vi "GetIMFreqs.vi"(6 "Legacy (f)?":bool, 8 "error in (no error)":errorcluster) -> (0 "error out":errorcluster, 2 "IMFreqs":dbl[](array[numeric]) format="%.2f")   [LabVIEW 2011]
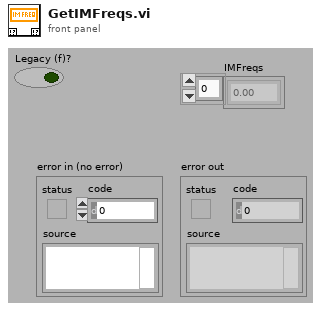
[diagram p1: front panel]
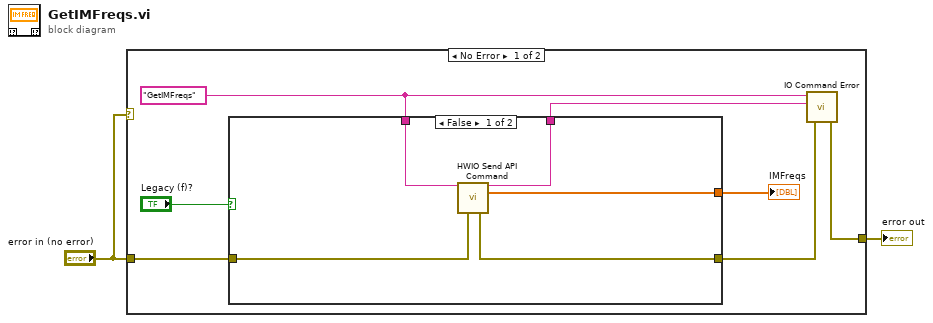
[diagram p0: block diagram]
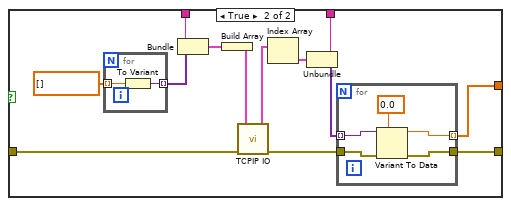
[diagram p2: hidden frame]
diagram:
  n1 = case shown="No Error" "error in (no error)" {
    tunnel: "error in (no error)" -> [w8 w35]
    tunnel: [w5 w35] -> w2
    frame No Error {
      w7 = "GetIMFreqs"
      n2 = case shown="False" "Legacy (f)?" {
        tunnel: [w12 w23] -> w9
        tunnel: w8 -> [w14 w21]
        tunnel: w7 -> [w10 w20]
        tunnel: [w13 w19] -> w6
        tunnel: [w11 w18] -> w4
        frame False {
          n3 = call "HWIO Send API Command.vi"("Action"=w10, "error in (no error)"=w14) -> ("Action out"=w11:string, "Double out"=w12:dbl[], "error out"=w13:errorcluster)  [unwired: 6 in, 5 out]
        }
        frame True {
          n4 = for {
            tunnel: [w34] -> w26 mode=indexing
            tunnel: dbl[] [] -> [w33] mode=indexing
            n5 = To Variant(anything=w33) -> (Variant=w34:variant)
          }
          n6 = Bundle(w20, w26) -> (w27:cluster{string, variant[]})  [unwired: 1 out]
          n7 = Build Array(w27) -> (w17:cluster{string, variant[]}[])
          n8 = call "TCPIP IO.vi"("error in (no error)"=w21, "Commands"=w17) -> ("error out"=w22:errorcluster, "Responses"=w16:cluster{string, variant[]}[])  [unwired: 1 in, 3 out]
          n9 = Index Array(array=w16) -> (element=w15:cluster{string, variant[]})  [unwired: 1 in]
          n10 = Unbundle(w15) -> (w18:string, w24:variant[])
          n11 = for {
            tunnel: [w32] -> w19
            tunnel: w22 -> [w31]
            tunnel: w24 -> [w29] mode=indexing
            tunnel: [w28] -> w23 mode=indexing
            n12 = Variant To Data(error in=w31, type=0.0, Variant=w29) -> (data=w28:dbl, error out=w32:errorcluster)
          }
        }
      }
      "IMFreqs" <- w9
      n13 = call "IO Command Error.vi"("error in (no error)"=w6, "Command Returned (\"\")"=w4, "Command Sent (\"\")"=w7) -> ("error out"=w5:errorcluster)  [unwired: 4 out]
    }
    frame Error {
    }
  }
  "error out" <- w2
